vi "LVM_LECTURA.vi"() -> ()   [LabVIEW 2020]
panel:
  out "Temp":dbl
  in  "stop":bool
  out "Datos":dynamicdata(graph)
  out "Alarma":bool
  out "Limite":dbl
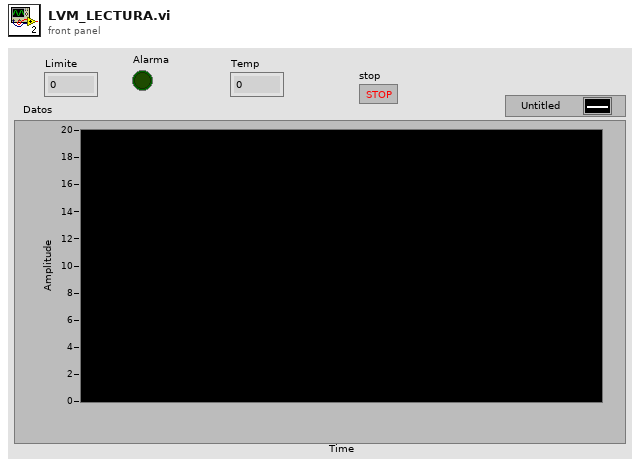
[diagram p1: front panel]
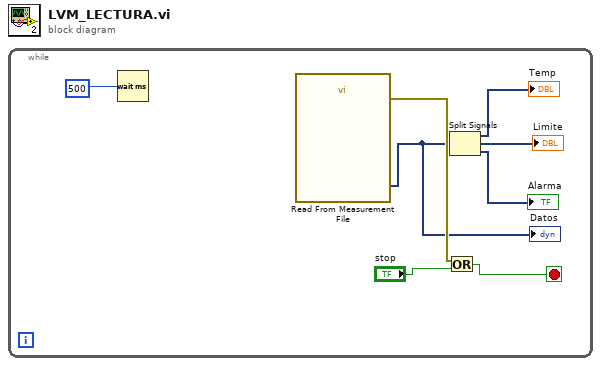
[diagram p0: block diagram]
diagram:
  n1 = while {
    stop <- w7 stop-if-true
    n2 = Wait (ms)(milliseconds to wait=u32 500 ("millisecond timer value")) -> ()  [unwired: 1 out]
    n3 = call "Read From Measurement File"() -> ("error out"=w5:errorcluster, "Signals"=w3:dynamicdata)  [unwired: 6 in, 4 out]
    "Datos" <- w3
    n4 = Or(x=w5, y="stop") -> (x .or. y?=w7:bool)
    n5 = Split Signals(w3) -> (→"Temp":dynamicdata, →"Limite":dynamicdata, →"Alarma":dynamicdata)  [unwired: 3 in]
  }
